vi "Task Unavailable Error to Warning.vi"(8 "error in (no error)":errorcluster) -> (0 "error out":errorcluster)   [LabVIEW 2017, in "Futures.lvlib" / "Task.lvclass"]
doc: "Downgrade the unavailable error to a warning where this isn't critical."
uses:
  Task.lvclass
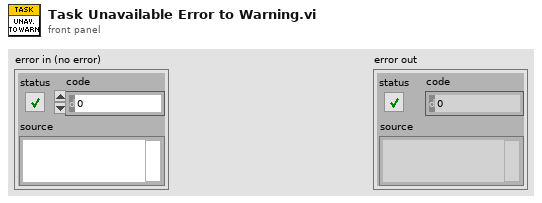
[diagram p1: front panel]
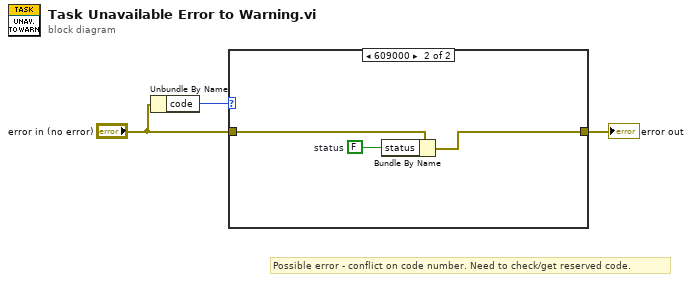
[diagram p0: block diagram]
diagram:
  # "Possible error - conflict on code number. Need to check/get reserved code."
  n1 = Unbundle By Name("error in (no error)") -> ("code"=w2:i32)
  n2 = case shown="609000" w2 {
    tunnel: [w4 w6] -> w3
    tunnel: "error in (no error)" -> [w4 w7]
    frame 0, Default {
    }
    frame 609000 {
      w5 = FALSE  # status
      n3 = Bundle By Name(cluster=w7, "status"=w5) -> (w6:errorcluster)
    }
  }
  "error out" <- w3
